vi "REPORT.Main Info.vi"(5 "Delimiter":string, 10 "CSV In":string, 11 "Test IN":T1 {"Test Registros"."Read W/R" format="%04x"; "Test Registros"."Pattern W/R" format="%04x"; "Test Registros"."Read Default" format="%04x"; "Test Registros"."Pattern Default" format="%04x"}) -> (2 "CSV Out":string)   [LabVIEW 2009]
uses:
  Test_result.ctl
  test_result fvasic.ctl
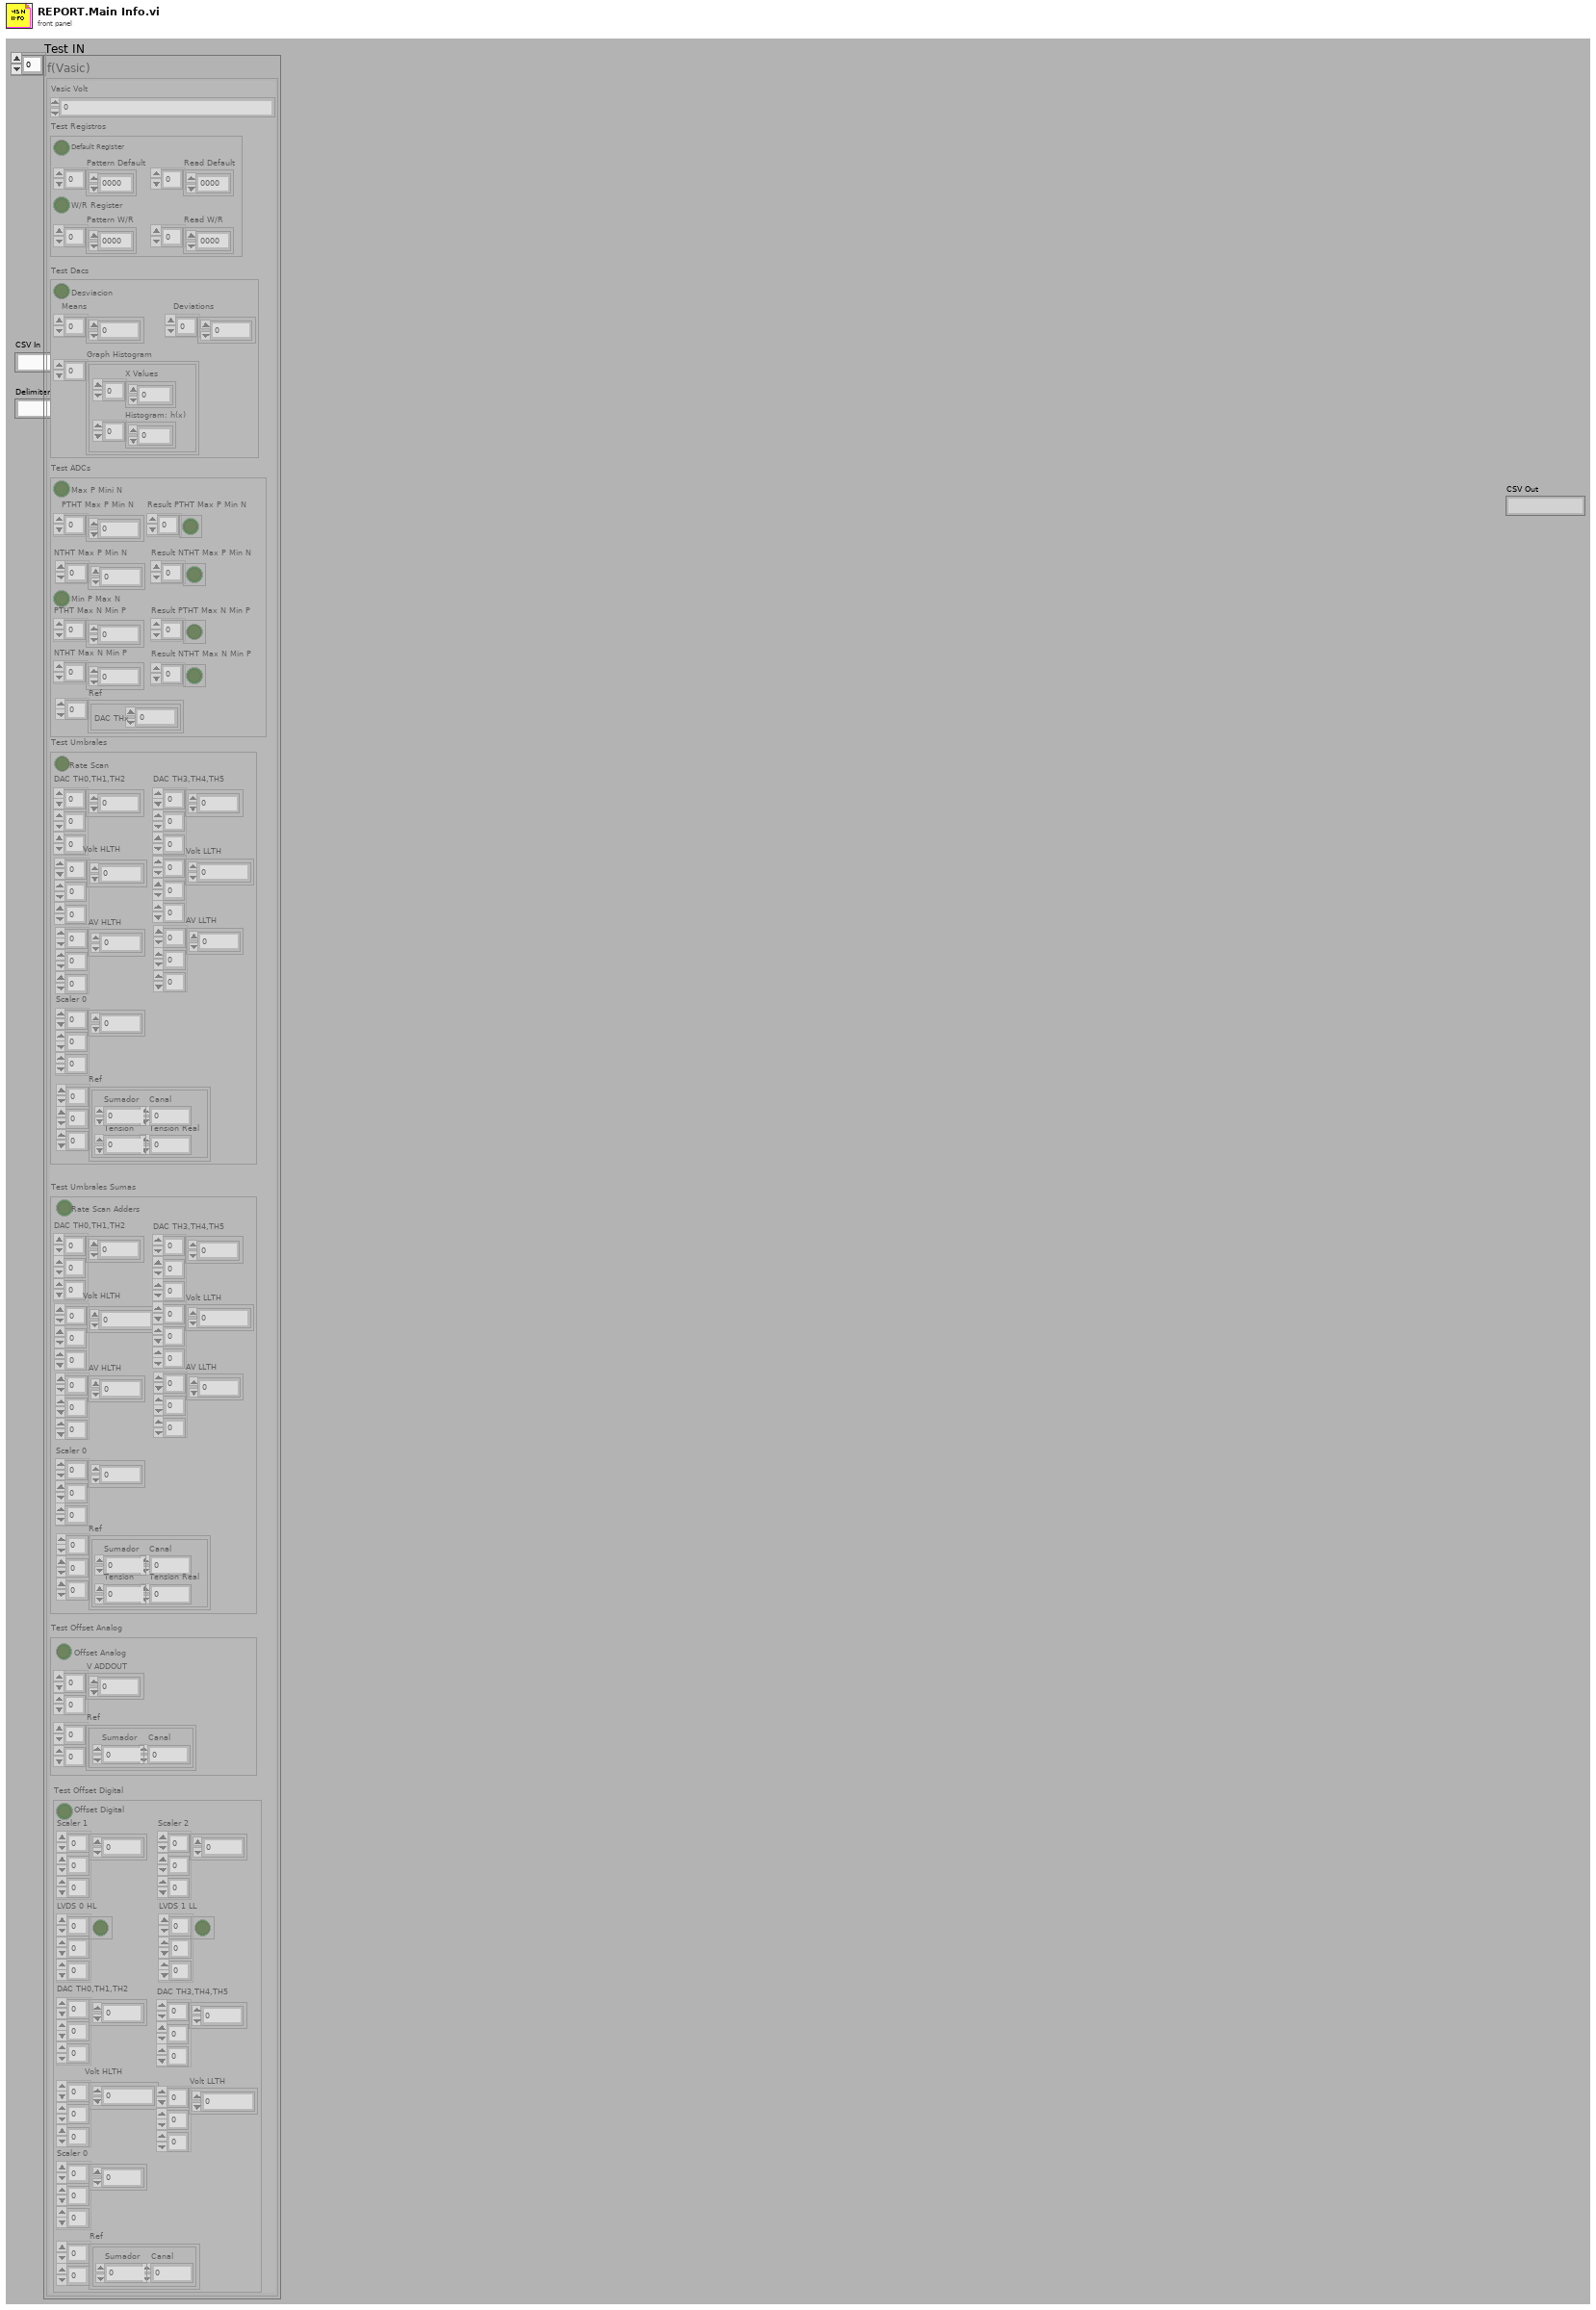
[diagram p1: front panel]
types:
  T1 = typedef "Test_result.ctl" = T2[]
  T2 = typedef "test_result fvasic.ctl" = cluster{"Vasic Volt":i32, "Test Registros":cluster{"Default Register":bool, "Pattern Default":u16[], "Read Default":u16[], "W/R Register":bool, "Pattern W/R":u16[], "Read W/R":u16[]}, "Test Dacs":cluster{"Desviacion":bool, "Means":dbl[], "Deviations":dbl[], "Graph Histogram":cluster{"X Values":dbl[], "Histogram: h(x)":i32[]}[]}, "Test ADCs":cluster{"Max P Mini N":bool, "PTHT Max P Min N":dbl[], "Result PTHT Max P Min N":bool[], "NTHT Max P Min N":dbl[], "Result NTHT Max P Min N":bool[], "Min P Max N":bool, "PTHT Max N Min P":dbl[], "Result PTHT Max N Min P":bool[], "NTHT Max N Min P":dbl[], "Result NTHT Max N Min P":bool[], "Ref":cluster{"DAC THx":u8}[]}, "Test Umbrales":cluster{"Rate Scan":bool, "DAC TH0,TH1,TH2":u16[][][], "Volt HLTH":dbl[][][], "AV HLTH":dbl[][][], "DAC TH3,TH4,TH5":u16[][][], "Volt LLTH":dbl[][][], "AV LLTH":dbl[][][], "Scaler 0":u16[][][], "Ref":cluster{"Sumador":u8, "Canal":u8, "Tension":u8, "Tension Real":dbl}[][][]}, "Test Umbrales Sumas":cluster{"Rate Scan Adders":bool, "DAC TH0,TH1,TH2":u16[][][], "Volt HLTH":dbl[][][], "AV HLTH":dbl[][][], "DAC TH3,TH4,TH5":u16[][][], "Volt LLTH":dbl[][][], "AV LLTH":dbl[][][], "Scaler 0":u16[][][], "Ref":cluster{"Sumador":u8, "Canal":u8, "Tension":u8, "Tension Real":dbl}[][][]}, "Test Offset Analog":cluster{"Offset Analog":bool, "V ADDOUT":dbl[][], "Ref":cluster{"Sumador":u8, "Canal":u8}[][]}, "Test Offset Digital":cluster{"Offset Digital":bool, "Scaler 1":u16[][][], "LVDS 0 HL":bool[][][], "DAC TH0,TH1,TH2":u16[][][], "Volt HLTH":dbl[][][], "Scaler 2":u16[][][], "LVDS 1 LL":bool[][][], "DAC TH3,TH4,TH5":u16[][][], "Volt LLTH":dbl[][][], "Scaler 0":u16[][][], "Ref":cluster{"Sumador":u8, "Canal":u8}[][]}}
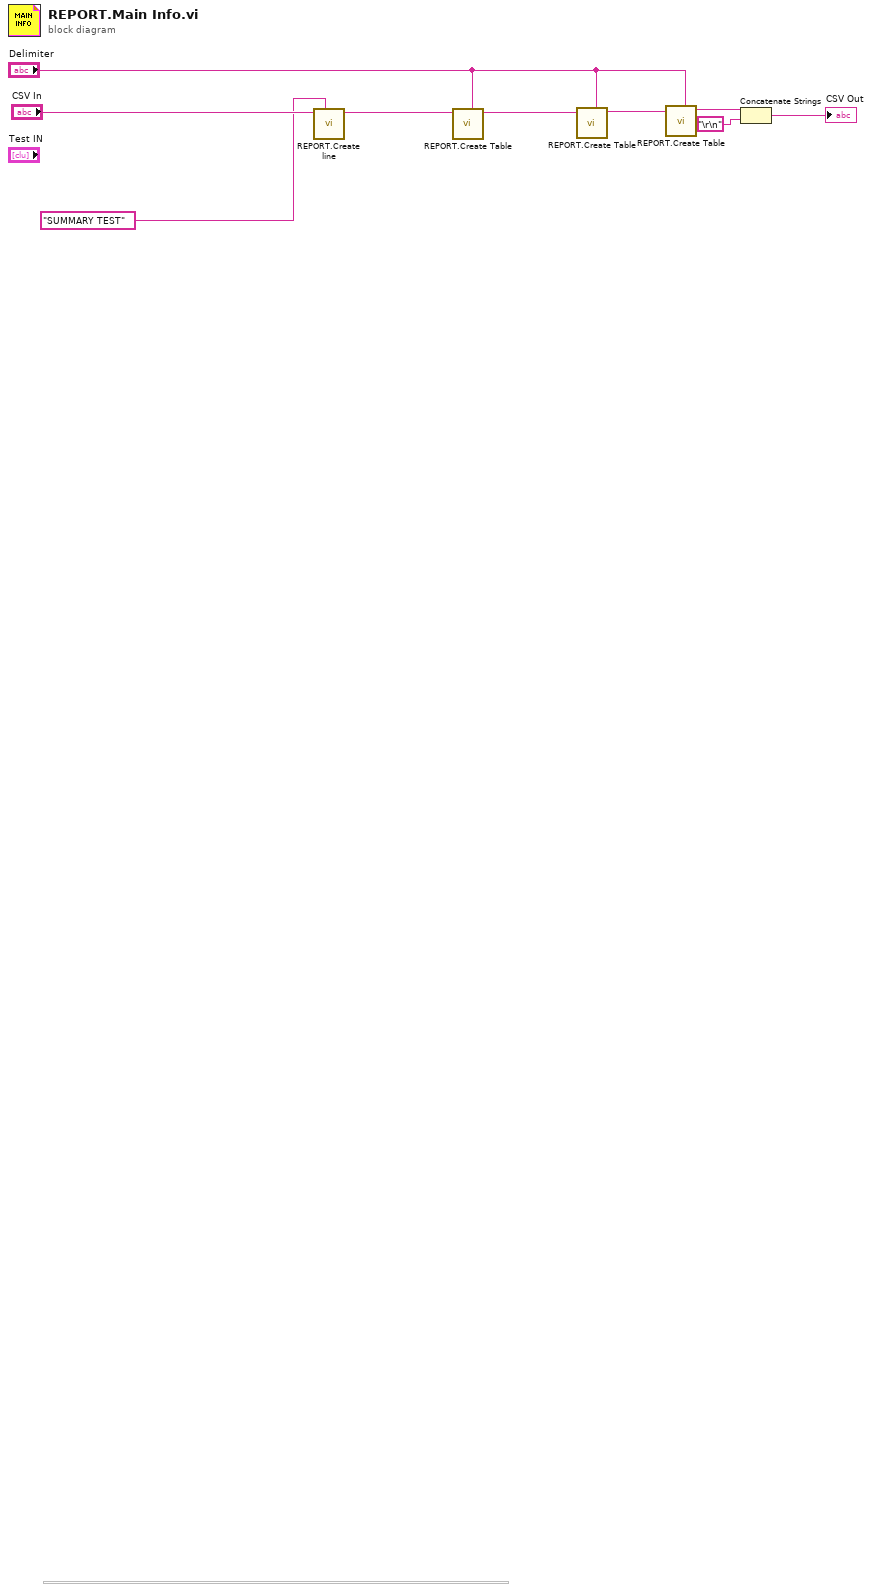
[diagram p0: block diagram]
diagram:
  n1 = call "REPORT.Create line.vi"("Secction"="SUMMARY TEST", "Text In"="CSV In") -> ("Text Out"=w7:string)  [unwired: 9 in]
  n2 = call "REPORT.Create Table.vi"("delimiter (Tab)"="Delimiter", "Text In"=w7) -> ("Text Out"=w9:string)  [unwired: 6 in, 1 out]
  n3 = call "REPORT.Create Table.vi"("delimiter (Tab)"="Delimiter", "Text In"=w9) -> ("Text Out"=w4:string)  [unwired: 6 in, 1 out]
  n4 = call "REPORT.Create Table.vi"("delimiter (Tab)"="Delimiter", "Text In"=w4) -> ("Text Out"=w2:string)  [unwired: 6 in, 1 out]
  n5 = Concatenate Strings(w2, "\r\n") -> (→"CSV Out":string)
